vi "0-Do Overlays.vi"(0 "Image Reference\nand Descriptor":cluster{"Image Out":T1, "Image Descriptor":T2} {"Image Descriptor"."Upper-Left Corner Coordinates"."North" format="%#_10f"; "Image Descriptor"."Upper-Left Corner Coordinates"."East" format="%#_8f"}, 1 "Missions":refnum<class "Mission.lvclass">[](array[class]), 5 "Waypoints":T7, 7 "Current Waypoint #":T6, 9 "Heading":T4 format="%05.1f", 11 "Sail Position":T5=0.5, 12 "Robot UTM Location":T3 {"North" format="%#_10f"; "East" format="%#_8f"}) -> (4 "Image out":T1)   [LabVIEW 2011]
doc: "Overlays waypoints and a boat icon on the image."
uses:
  <vilib>/vision/Image Controls.llb/IMAQ Image.ctl
  0x2-OCU-Think Comm/0x2 Typedefs/Waypoints List.ctl
  2-Think/2 Classes/Waypoint/Waypoint.lvclass
  0x2-OCU-Think Comm/0x2 Typedefs/Current Waypoint.ctl
  2-Think/2 Typedefs/sail setpt.ctl
  2-Think/2 Typedefs/heading.ctl
  2-Think/2 Typedefs/UTM Location.ctl
  0-Image Descriptor.ctl
  2-Think/2 Classes/Mission/Mission.lvclass
panel:
  out "Boat Outside Img":bool
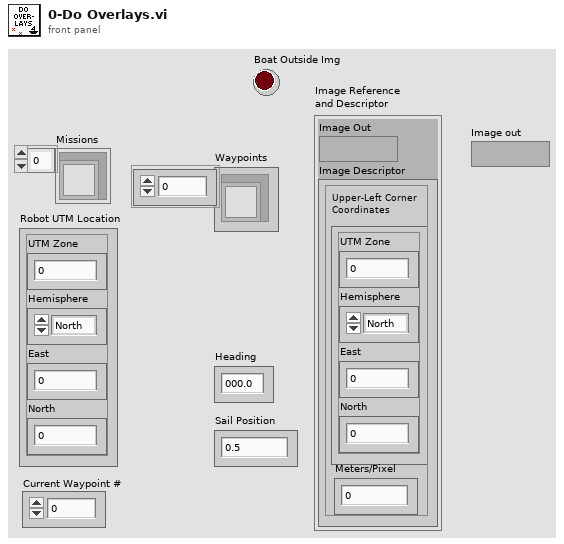
[diagram p1: front panel]
types:
  T1 = typedef "IMAQ Image.ctl" = refnum<image>
  T2 = typedef "0-Image Descriptor.ctl" = cluster{"Upper-Left Corner Coordinates":T3, "Meters/Pixel":dbl}
  T3 = typedef "UTM Location.ctl" = cluster{"UTM Zone":dbl, "Hemisphere":enum16{"North", "South"}, "East":dbl, "North":dbl}
  T4 = typedef "heading.ctl" = dbl
  T5 = typedef "sail setpt.ctl" = dbl
  T6 = typedef "Current Waypoint.ctl" = i32
  T7 = typedef "Waypoints List.ctl" = refnum<class "Waypoint.lvclass">[]
  T8 = typedef "Overlay References.ctl" = cluster{"Boat Icon, Unroatated":T1, "Boat Icon, Rotated":T1, "Sail Icon, Unrotated":T1, "Sail Icon, Rotated":T1}
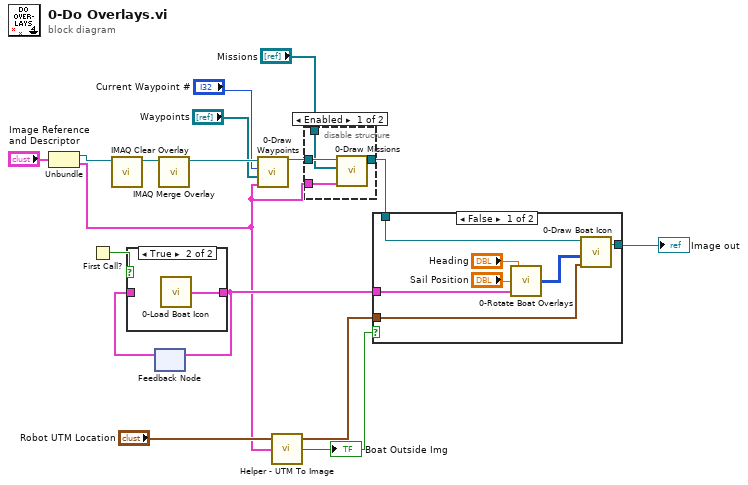
[diagram p0: block diagram]
diagram:
  n1 = Unbundle("Image Reference\nand Descriptor") -> ("Image Out"=w5:T1, "Image Descriptor"=w4:T2)
  n2 = First Call?() -> (First Call?: T/F=w14:bool)
  n3 = call "IMAQ Clear Overlay"("Image"=w5) -> ("Image Out"=w17:T1)  [unwired: 2 in, 8 out]
  n4 = feedback #1() -> (w12:T8)  [unwired: 1 in]
  n5 = case shown="True" w14 {
    tunnel: [w18 w19] -> w13
    tunnel: w12 -> [w18 _]
    frame False {
      # "image already\nloaded"
    }
    frame True {
      n6 = call "0-Load Boat Icon.vi"() -> ("Overlay References Out"=w19:T8)  [unwired: 1 in]
    }
  }
  n7 = feedback-in #1(w13) -> ()
  n8 = call "IMAQ Merge Overlay"("Image Src"=w17) -> ("Image Dst Out"=w15:T1)  [unwired: 4 in, 6 out]
  n9 = call "0-Draw Waypoints.vi"("Image Descriptor"=w4, "Waypoints List"="Waypoints", "Current Waypoint #"="Current Waypoint #", "Image In"=w15) -> ("Image Out"=w3:T1)  [unwired: 2 in, 1 out]
  n10 = call "Helper - UTM To Image.vi"("Image Descriptor"=w4, "UTM Location"="Robot UTM Location") -> ("Coordinate Outside Image"=w9:bool, "Pixel Coordinates"=w8:cluster{"X":i32, "Y":i32})  [unwired: 1 in, 1 out]
  "Boat Outside Img" <- w9
  n11 = disable-structure shown="Enabled" {
    disable-tunnel: w4 -> [w23 _]
    disable-tunnel: w3 -> [w22 w24]
    disable-tunnel: [w21 w24] -> w2
    disable-tunnel: "Missions" -> [w20 _]
    frame Enabled {
      n12 = call "0-Draw Missions.vi"("Image Descriptor"=w23, "Missions"=w20, "Image In"=w22) -> ("Image Out"=w21:T1)  [unwired: 4 in]
    }
    frame Disabled {
    }
  }
  n13 = case shown="False" w9 {
    tunnel: [w31 w32] -> w16
    tunnel: w2 -> [w30 w32]
    tunnel: w8 -> [w29 _]
    tunnel: w13 -> [w27 _]
    frame False {
      n14 = call "0-Rotate Boat Overlays.vi"("Overlay References In"=w27, "Sail Position"="Sail Position", "Heading"="Heading") -> ("Rotated Boat Icon Bitmap Out"=w28:u32[][])  [unwired: 1 in, 1 out]
      n15 = call "0-Draw Boat Icon.vi"("Position"=w29, "Boat Bitmap"=w28, "Image In"=w30) -> ("Image Out"=w31:T1)  [unwired: 4 out]
    }
    frame True {
      # "don't draw\nif boat\noutside\nimage"
    }
  }
  "Image out" <- w16
